vi "6.vi"() -> ()   [LabVIEW 2012]
panel:
  out "Real 2":dbl
  in  "Real":dbl
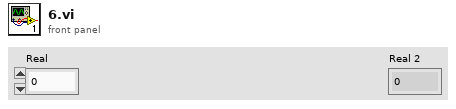
[diagram p1: front panel]
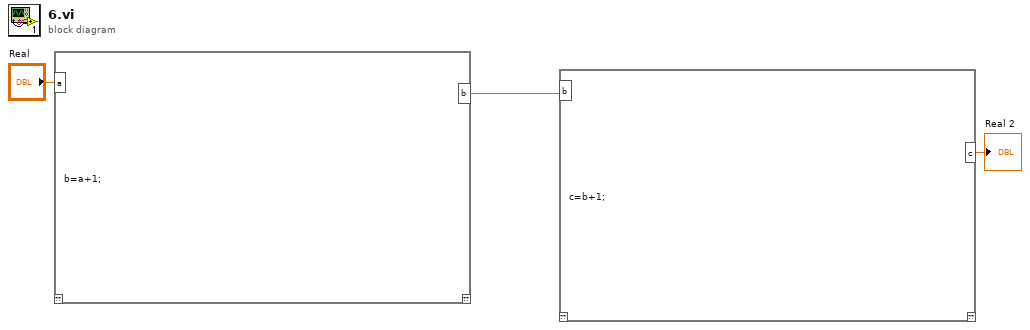
[diagram p0: block diagram]
diagram:
  n1 = script code="b=a+1;"("a"="Real") -> ("b"=w2:dbl)  [unwired: 1 in, 1 out]
  n2 = script code="c=b+1;"("b"=w2) -> ("c"=→"Real 2":dbl)  [unwired: 1 in, 1 out]
